vi "hmi_status.vi"(7 "hmi_references":T2, 8 "error in (no error)":errorcluster, 10 "action":T1, 11 "build_spec.build_spec_name":string) -> (0 "error out":errorcluster)   [LabVIEW 2015, in "lv-build-interface.lvlib"]
uses:
  lv-build-interface.lvlib
  _controls/hmi_references.ctl
  _controls/action.ctl
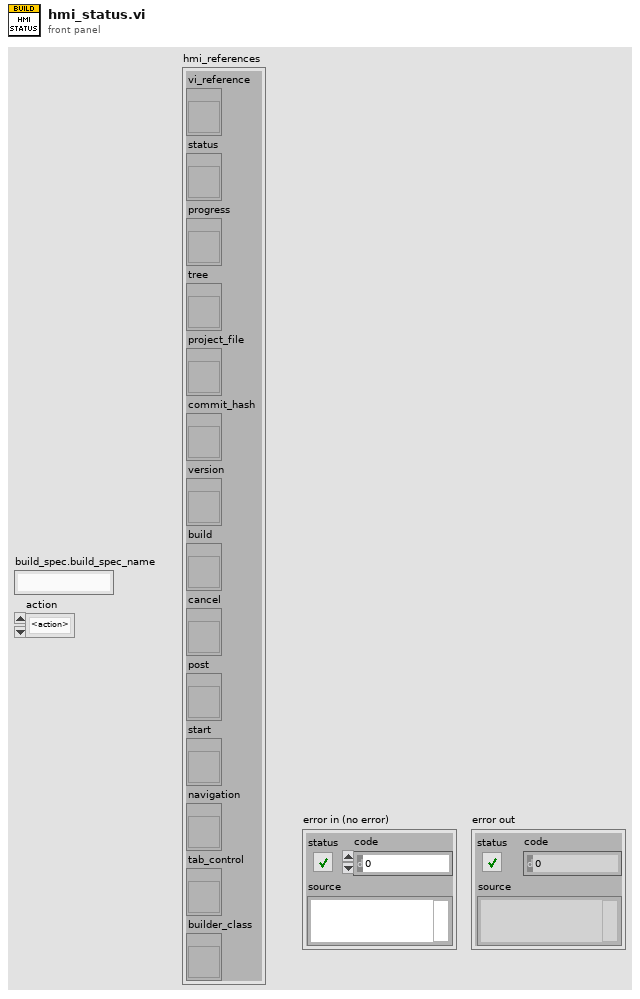
[diagram p1: front panel]
types:
  T1 = typedef "lv-build-interface.lvlib/action.ctl" = enum16{"<action>", "build", "post", "deploy", "<null>"}
  T2 = typedef "lv-build-interface.lvlib/hmi_references.ctl" = cluster{"vi_reference":refnum<vi>, "status":refnum<vi>, "progress":refnum<vi>, "tree":refnum<vi>, "project_file":refnum<vi>, "commit_hash":refnum<vi>, "version":refnum<vi>, "build":refnum<vi>, "cancel":refnum<vi>, "post":refnum<vi>, "start":refnum<vi>, "navigation":refnum<vi>, "tab_control":refnum<vi>, "builder_class":refnum<vi>}
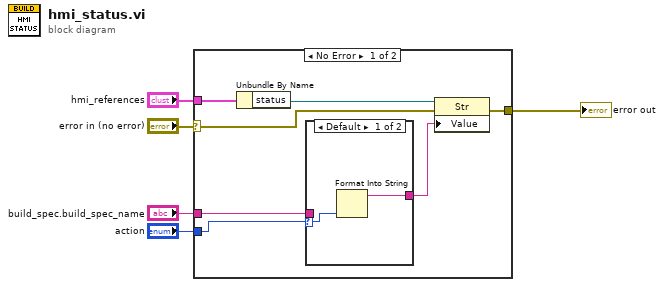
[diagram p0: block diagram]
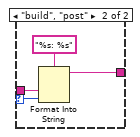
[diagram p2: hidden frame]
diagram:
  n1 = case shown="No Error" "error in (no error)" {
    selector: "error in (no error)" -> [w9 w19]
    tunnel: "hmi_references" -> [w12 _]
    tunnel: [w8 w19] -> w3
    tunnel: "build_spec.build_spec_name" -> [w7 _]
    tunnel: "action" -> [w6 _]
    frame No Error {
      n2 = Unbundle By Name(w12) -> ("status"=w11:refnum<vi>)
      n3 = case shown="Default" w6 {
        selector: w6 -> [w14 w16]
        tunnel: w7 -> [_ w17]
        tunnel: [w13 w15] -> w10
        frame Default {
          n4 = Format Into String(w14) -> (resulting string=w13:string)  [unwired: 3 in, 1 out]
        }
        frame "build", "post" {
          n5 = Format Into String(format string="%s: %s", w17, w16) -> (resulting string=w15:string)  [unwired: 2 in, 1 out]
        }
      }
      n6 = property class="Str"(reference=w11, error in=w9, "Value"=w10) -> (error out=w8:errorcluster)  [unwired: 1 out]
    }
    frame Error {
    }
  }
  "error out" <- w3
